vi "Acq Configure Transfer.vi"(0 "session in":refnum<class "Digitizer Control.lvclass">, 1 "host DMA buffer size (samples)":u32[](array[numeric]), 2 "host DMA buffer num of blocks":u32[](array[numeric]), 3 "host DMA buffer block size divisor (bytes)":u32[](array[numeric]), 4 "trigger delay tracking enable (F)":bool, 5 "error in (no error)":errorcluster, 7 "disable DRAM FIFO (F)":bool[](array[boolean]), 9 "enable bit packing (F)":bool[](array[boolean])) -> (13 "sample size (bits)":i32[](array[numeric]), 14 "session out":refnum<class "Digitizer Control.lvclass">, 15 "actual host DMA buffer size (samples)":u32[](array[numeric]), 16 "actual host DMA buffer size (elements)":u32[](array[numeric]), 17 "transfer quantum size (samples)":u64[](array[numeric]), 18 "transfer quantum size (elements)":u64[](array[numeric]), 19 "error out":errorcluster)   [LabVIEW 2021, in "Digitizer Control.lvclass"]
doc: "Configures the acquisition waveform transfer parameters. Note that the transfer parameters can be configured only after the channel parameters are configured. Use the <B>Acq Configure Start Trigger.vi</B> to configure the start trigger, and the <B>Acq Configure Channel.vi</B> to configure the channel parameters. Once the acquisition is configured, use the <B>Acq Initiate.vi</B> to initiate an acquisition, then use the <B>Acq Fetch Waveform.vi</B> to fetch the acquired samples. Use the <B>Acq Get Status.vi</B> to check the acquisition status and the <B>Acq Stop.vi</B> to stop an acquisition.\n\nInputs:\n\n<B>session in</B>: The device session.\n\n<B>host DMA buffer size (samples)</B>: The desired host DMA buffer size given in number of samples. This input is an array, the n-th element corresponds to the n-th channel.\n\n<B>host DMA buffer num of blocks</B>, <B>host DMA buffer block size divisor (bytes)</B>: Use these inputs to apply size constraints on the host DMA buffer size. The size of the allocated host DMA buffer will be a multiple of <B>host DMA buffer num of blocks</B>, and dividing the size of the allocated host DMA buffer by <B>host DMA buffer num of blocks</B> results in a size which is an integer multiple of the sample size, and in bytes is an integer multiple of the <B>host DMA buffer block size divisor (bytes)</B>. These inputs are arrays, the n-th element of an array corresponds to the n-th channel.\n\n<B>trigger delay tracking enable</B>: A true on this input enables the recording of the delay between the device receiving a trigger and starting the acquisition. TClk synchronized acquisitions have an inherent trigger response latency that is between 1-2 TClk periods. The latency can be compensated by acquiring additional pre-trigger samples and keeping only latency worth of the additional pre-trigger samples. When using TClk synchronization, use the <B>Acq Configure Pretrigger Period.vi</B> on all devices to enable the acquisition of the additional pre-trigger samples, and enable this option on the master device to record the trigger response latency. When fetching a record, use the <B>Acq Fetch Trigger Delay.vi</B> on the master device to fetch the recorded delay value and the number of samples to remove from the beginning of the record to align the record with the trigger.\n\n<B>disable DRAM FIFO</B>: Array of booleans, a true in the n-th element of this array disables the use of the DRAM memory available on the device for buffering the samples acquired on the n-th channel.\n\n<B>enable bit packing</B>: Array of booleans, a true in the n-th element of this array enables bit packing for the n-th channel. The device always transfers 16-bit data elements to the host. If bit packing is disabled then the device transfers 16-bit samples to the host, one sample in each data element. If bit packing is enabled then the device transfers 12-bit samples packed into 16-bit data elements to the host (4 samples per 3 data elements).\n\nOutputs:\n\n<B>session out</B>: The device session passed on the <B>session in</B> input.\n\n<B>actual host DMA buffer size (samples)</B>: The actual host DMA buffer size given in number of samples. This output is an array, the n-th element corresponds to the n-th channel.\n\n<B>actual host DMA buffer size (elements)</B>: The actual host DMA buffer size given in number of elements. This output is an array, the n-th element corresponds to the n-th channel.\n\n<B>transfer quantum size (samples)</B>: The smallest number of samples whose size is an integer multiple of the sample transfer interface width. Transferring quantum size multiple samples allows the device to transfer integer number of samples without waiting for further samples to complete the transfer. This output is an array, the n-th element corresponds to the n-th channel.\n\n<B>transfer quantum size (elements)</B>: The number of elements required to transfer <B>transfer quantum size (samples)</B> number of samples. This output is an array, the n-th element corresponds to the n-th channel.\n\n<B>sample size (bits)</B>: The size of a sample, given in bits, the FPGA Target is using when transferring the samples. This output is an array, the n-th element corresponds to the n-th channel."
uses:
  Digitizer Control.lvclass
  Digitizer Control.lvclass/Digitizer Control.ctl
  <vilib>/Utility/error.llb/Error Cluster From Error Code.vi
  <vilib>/rvi/errors/niLvFpgaAdjustHostInterfaceError.vi
  <vilib>/rvi/interface/common/niFpgaWaitOnOcc.vi
  <vilib>/ErrorRing/Error Ring.xnode
  <vilib>/rvi/interface/nirviReadWriteControl/nirviReadWriteControl.xnode
  <vilib>/rvi/interface/nirviMethod/nirviMethod.xnode
  <instrlib>/_niInstr/Streaming/v1/Host/niInstr Streaming v1 Host.lvlib
  <vilib>/rvi/errors/niLvFpgaMergeErrorWithErrorCode.vi
  <vilib>/FPGAPlugInAG/Dynamic/niLvFpga_StartFifo_Dynamic.vi
  <vilib>/FPGAPlugInAG/Dynamic/niLvFpga_ConfigureFifo_Dynamic.vi
  <vilib>/gmath/NI_Gmath.lvlib
  NiFpgaLv.dll
  <vilib>/rvi/interface/Simulation/niFpgaSimulationCallBeginRW.vi
  <vilib>/FPGAPlugInAG/Dynamic/niLvFpga_StopFifo_Dynamic.vi
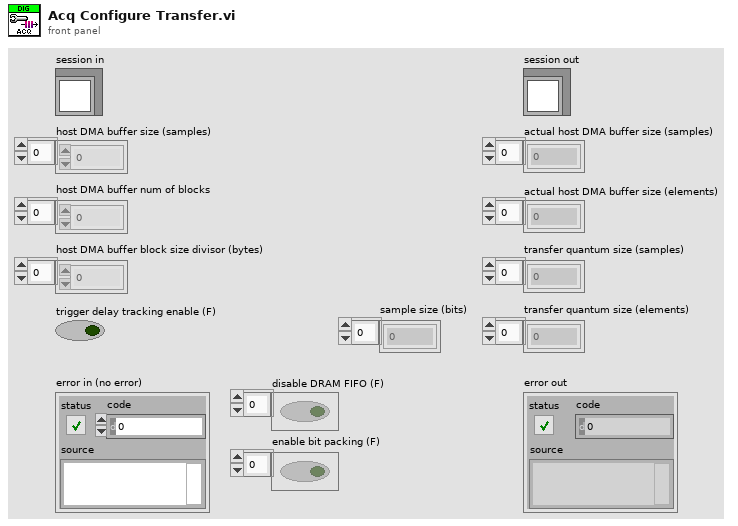
[diagram p1: front panel]
types:
  T1 = typedef "Digitizer Control.lvclass/Acq Session Data.ctl" = cluster{"ADC sampling rate":dbl, "SCTL rate":dbl, "DMA element size (bits)":i32, "sample size (bits)":i32[], "DMA/memory interface width (DMA elements)":i32, "transfer size (bits)":i32[], "stream instance":i32[], "trigger instance":u32, "group delay (s)":dbl, "data delay (s)":dbl, "target delay (s)":dbl, "trigger tracking enabled":bool, "channel configured":bool, "enabled channels":bool[], "transfer configured":bool, "dsp bypass":bool, "fractional decimator input rate":dbl, "fractional decimator output rate":dbl, "sample scale factor":dbl[], "memory size":u64[], "FIFO size":u64}
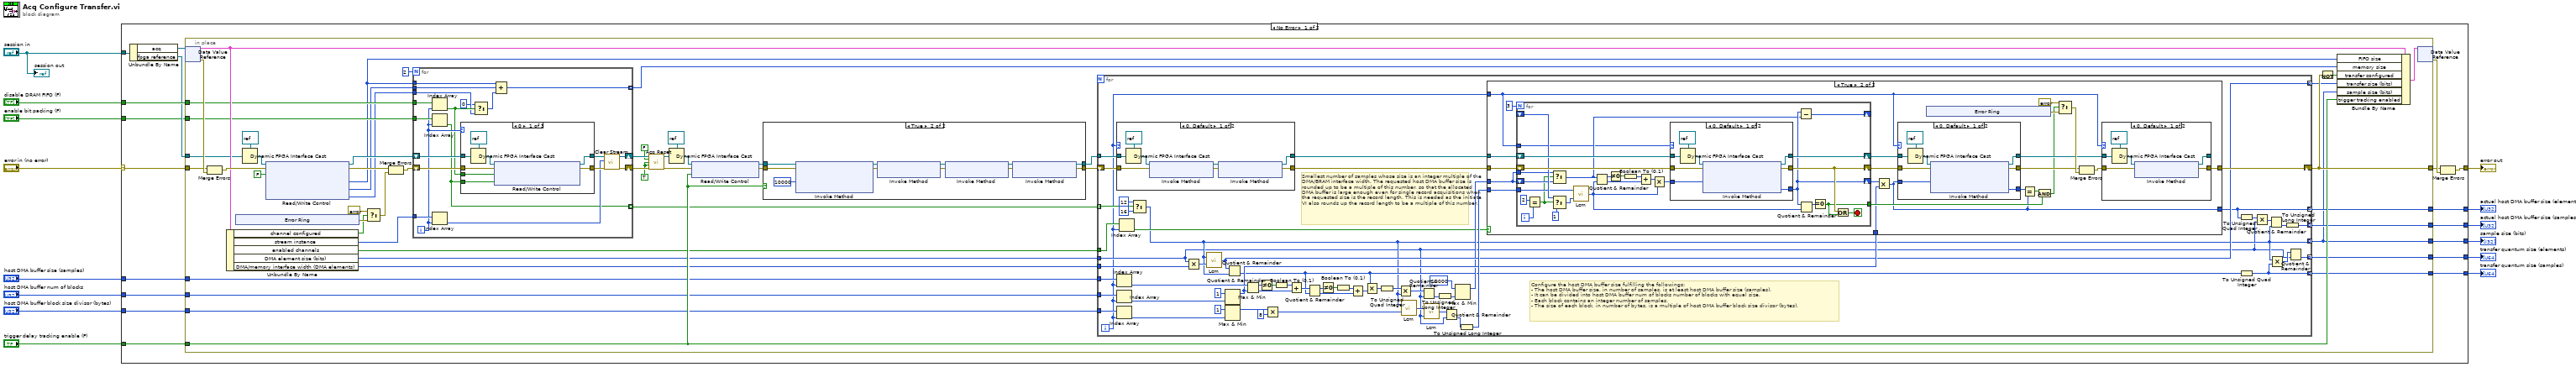
[diagram p0: block diagram]
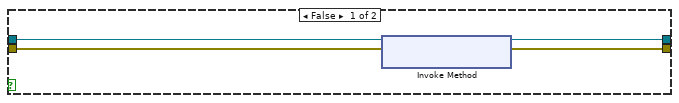
[diagram p2: hidden frame]
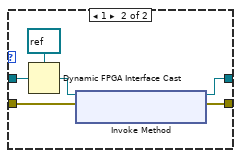
[diagram p4: hidden frame]
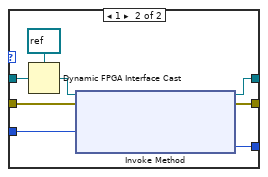
[diagram p5: hidden frame]
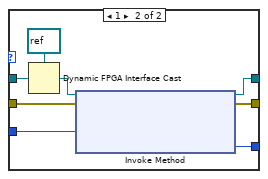
[diagram p6: hidden frame]
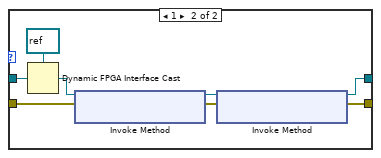
[diagram p7: hidden frame]
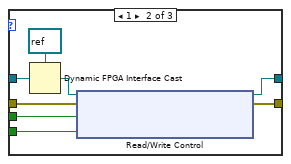
[diagram p8: hidden frame]
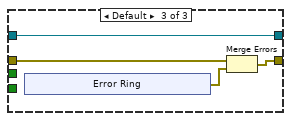
[diagram p9: hidden frame]
diagram:
  n1 = case shown="No Error" "error in (no error)" {
    selector: "error in (no error)" -> [w31 w322]
    tunnel: "session in" -> [w24 _]
    tunnel: [w26 w322] -> w13
    tunnel: "host DMA buffer size (samples)" -> [w30 _]
    tunnel: "disable DRAM FIFO (F)" -> [w29 _]
    tunnel: [w28 _] -> w10
    tunnel: [w25 _] -> w9
    tunnel: "enable bit packing (F)" -> [w21 _]
    tunnel: "trigger delay tracking enable (F)" -> [w20 _]
    tunnel: "host DMA buffer num of blocks" -> [w19 _]
    tunnel: "host DMA buffer block size divisor (bytes)" -> [w18 _]
    tunnel: [w17 _] -> w3
    tunnel: [w16 _] -> w2
    tunnel: [w15 _] -> w1
    frame No Error {
      n2 = Unbundle By Name(w24) -> ("acq"=w23:refnum<data-value>, "fpga reference"=w22:refnum<k20>)
      n3 = in-place {
        in-place-border: [w84] -> w27
        in-place-border: w31 -> [w70]
        in-place-border: w30 -> [w65]
        in-place-border: w29 -> [w42]
        in-place-border: [w66] -> w28
        in-place-border: [w67] -> w25
        in-place-border: w22 -> [w62]
        in-place-border: w21 -> [w59]
        in-place-border: w20 -> [w83]
        in-place-border: w19 -> [w44]
        in-place-border: w18 -> [w43]
        in-place-border: [w36] -> w17
        in-place-border: [w34] -> w16
        in-place-border: [w33] -> w15
        w53 = TRUE
        n4 = in-place-dvr #1(w23) -> (w74:T1, w73:errorcluster)
        n5 = Merge Errors(w70, w73) -> (w79:errorcluster)
        n6 = Unbundle By Name(w74) -> ("channel configured"=w61:bool, "stream instance"=w58:i32[], "enabled channels"=w55:bool[], "DMA element size (bits)"=w63:i32, "DMA/memory interface width (DMA elements)"=w64:i32)
        n7 = xnode "Error Ring"() -> ("error out"=w77:errorcluster)
        n8 = Dynamic FPGA Interface Cast(Session In=refnum<k20> refnum ("FPGA Interface"), Type=w62) -> (Session Out=w71:refnum<k20>)
        n9 = xnode "Read/Write Control"("FPGA VI Reference In"=w71, "error in"=w79, "acq.stream.start enable"=FALSE) -> ("FPGA VI Reference Out"=w60:refnum<k20>, "error out"=w78:errorcluster, "acq.wfm.FIFO size"=w38:u64, "acq.wfm.memory FIFO size"=w40:u64, "acq.wfm.memory DRAM size"=w39:u64)
        n10 = Select(t=errorcluster {"status"=FALSE, "code"=0, "source"=""}, s=w61, f=w77) -> (s? t:f=w75:errorcluster)
        n11 = Merge Errors(w78, w75) -> (w80:errorcluster)
        n12 = for {
          N: 2 -> [_]
          tunnel: w59 -> [w287]
          tunnel: w42 -> [w286]
          tunnel: w58 -> [w285]
          shift-right: [w291] -> w81
          shift-left: w80 -> [w289]
          tunnel: [w280] -> w56 mode=indexing
          shift-right: [w284] -> w82
          shift-left: w60 -> [w288]
          tunnel: w40 -> [w275]
          tunnel: w39 -> [w278]
          tunnel: w38 -> [w276]
          tunnel: [w273] -> w37 mode=indexing
          i -> [w281]
          n13 = Index Array(array=w286, index=w281) -> (element=w279:bool)
          n14 = Index Array(array=w287, index=w281) -> (element=w280:bool)
          n15 = Index Array(array=w285, index=w281) -> (element=w282:i32)
          n16 = case shown="0" w281 {
            tunnel: w288 -> [w297 w307 w311]
            tunnel: w289 -> [w299 w306 w310]
            tunnel: w279 -> [w296 w305 _]
            tunnel: w280 -> [w295 w304 _]
            tunnel: [w298 w301 w309] -> w290
            tunnel: [w292 w300 w311] -> w283
            frame 0 {
              n17 = Dynamic FPGA Interface Cast(Session In=refnum<k20> refnum ("FPGA Interface"), Type=w297) -> (Session Out=w293:refnum<k20>)
              n18 = xnode "Read/Write Control"("FPGA VI Reference In"=w293, "error in"=w299, "acq.wfm.bypass DRAM FIFO 0"=w296, "acq.wfm.enable bit packing 0"=w295) -> ("FPGA VI Reference Out"=w292:refnum<k20>, "error out"=w298:errorcluster)
            }
            frame 1 {
              n19 = Dynamic FPGA Interface Cast(Session In=refnum<k20> refnum ("FPGA Interface"), Type=w307) -> (Session Out=w302:refnum<k20>)
              n20 = xnode "Read/Write Control"("FPGA VI Reference In"=w302, "error in"=w306, "acq.wfm.bypass DRAM FIFO 1"=w305, "acq.wfm.enable bit packing 1"=w304) -> ("FPGA VI Reference Out"=w300:refnum<k20>, "error out"=w301:errorcluster)
            }
            frame Default {
              n21 = xnode "Error Ring"() -> ("error out"=w308:errorcluster)
              n22 = Merge Errors(w310, w308) -> (w309:errorcluster)
            }
          }
          n23 = Select(t=u64 0, s=w279, f=w278) -> (s? t:f=w274:u64)
          n24 = Compound Arithmetic op=ADD(w276, w275, w274) -> (w273:u64)
          n25 = call <instrlib>:"Clear Stream.vi"("error in (no error)"=w290, "stream index"=w282, "refnum in"=w283) -> ("error out"=w291:errorcluster, "refnum out"=w284:refnum<k20>)  [unwired: 7 in]
        }
        n26 = call "Acq Reset.vi"("fpga reference in"=w82, "reset dsp"=FALSE, "reset stream control"=w53, "reset waveform streaming"=w53, "error in (no error)"=w81) -> ("fpga reference out"=w49:refnum<k20>, "error out"=w48:errorcluster)  [unwired: 9 in]
        n27 = Dynamic FPGA Interface Cast(Session In=refnum<k20> refnum ("FPGA Interface"), Type=w49) -> (Session Out=w47:refnum<k20>)
        n28 = xnode "Read/Write Control"("FPGA VI Reference In"=w47, "error in"=w48, "trigger.monitor enable"=w83) -> ("FPGA VI Reference Out"=w45:refnum<k20>, "error out"=w46:errorcluster)
        n29 = case shown="True" w83 {
          tunnel: w46 -> [w88 w99]
          tunnel: [w85 w90] -> w52
          tunnel: w45 -> [w87 w97]
          tunnel: [w86 w89] -> w51
          frame False {
            n30 = xnode "Invoke Method"("FPGA VI Reference In"=w87, "error in"=w88) -> ("FPGA VI Reference Out"=w86:refnum<k20>, "error out"=w85:errorcluster)
          }
          frame True {
            n31 = xnode "Invoke Method"("FPGA VI Reference In"=w97, "error in"=w99, "Requested Depth"=u32 10000) -> ("FPGA VI Reference Out"=w95:refnum<k20>, "error out"=w96:errorcluster)  [unwired: 1 out]
            n32 = xnode "Invoke Method"("FPGA VI Reference In"=w95, "error in"=w96) -> ("FPGA VI Reference Out"=w93:refnum<k20>, "error out"=w94:errorcluster)
            n33 = xnode "Invoke Method"("FPGA VI Reference In"=w93, "error in"=w94) -> ("FPGA VI Reference Out"=w91:refnum<k20>, "error out"=w92:errorcluster)
            n34 = xnode "Invoke Method"("FPGA VI Reference In"=w91, "error in"=w92) -> ("FPGA VI Reference Out"=w89:refnum<k20>, "error out"=w90:errorcluster)
          }
        }
        n35 = for {
          tunnel: [w154] -> w67 mode=indexing
          tunnel: [w112] -> w66 mode=indexing
          tunnel: w65 -> [w153]
          tunnel: w64 -> [w152]
          tunnel: w63 -> [w102]
          tunnel: [w114] -> w35 mode=indexing
          tunnel: w56 -> [w121] mode=indexing
          tunnel: [w104] -> w34 mode=indexing
          tunnel: w55 -> [w119]
          shift-right: [w157] -> w84
          shift-left: w52 -> [w155]
          tunnel: w51 -> [w156]
          tunnel: w44 -> [w110]
          tunnel: w43 -> [w108]
          tunnel: [w105] -> w36 mode=indexing
          tunnel: [w101] -> w33 mode=indexing
          i -> [w100]
          # "Smallest number of samples whose size is an integer multiple of the DMA/BRAM interface width. The requested host DMA buffer size is rounded up to be a multiple of this number, so that the allocated DMA buffer is large enough even for single record acquisitions when the requested size is the record length. This is needed as the initiate VI also rounds up the record length to be a multiple of this number."
          # "Configure the host DMA buffer size fulfilling the followings:\n- The host DMA buffer size, in number of samples, is at least host DMA buffer size (samples).\n- It can be divided into host DMA buffer num of blocks number of blocks with equal size.\n- Each block contains an integer number of samples.\n- The size of each block, in number of bytes, is a multiple of host DMA buffer block size divisor (bytes)."
          n36 = case shown="0, Default" w100 {
            tunnel: [w262 w270] -> w125
            tunnel: [w261 w269] -> w124
            tunnel: w156 -> [w258 w266]
            tunnel: w155 -> [w260 w268]
            frame 0, Default {
              n37 = Dynamic FPGA Interface Cast(Session In=refnum<k20> refnum ("FPGA Interface"), Type=w258) -> (Session Out=w257:refnum<k20>)
              n38 = xnode "Invoke Method"("FPGA VI Reference In"=w257, "error in"=w260) -> ("FPGA VI Reference Out"=w263:refnum<k20>, "error out"=w264:errorcluster)
              n39 = xnode "Invoke Method"("FPGA VI Reference In"=w263, "error in"=w264) -> ("FPGA VI Reference Out"=w261:refnum<k20>, "error out"=w262:errorcluster)
            }
            frame 1 {
              n40 = Dynamic FPGA Interface Cast(Session In=refnum<k20> refnum ("FPGA Interface"), Type=w266) -> (Session Out=w265:refnum<k20>)
              n41 = xnode "Invoke Method"("FPGA VI Reference In"=w265, "error in"=w268) -> ("FPGA VI Reference Out"=w271:refnum<k20>, "error out"=w272:errorcluster)
              n42 = xnode "Invoke Method"("FPGA VI Reference In"=w271, "error in"=w272) -> ("FPGA VI Reference Out"=w269:refnum<k20>, "error out"=w270:errorcluster)
            }
          }
          n43 = Index Array(array=w153, index=w100) -> (element=w123:u32)
          n44 = Index Array(array=w110, index=w100) -> (element=w109:u32)
          n45 = Index Array(array=w108, index=w100) -> (element=w107:u32)
          n46 = Index Array(array=w119, index=w100) -> (element=w111:bool)
          n47 = Select(t=12, s=w121, f=16) -> (s? t:f=w104:i32)
          n48 = Multiply(x=w102, y=w152) -> (x*y=w136:i32)
          n49 = call <vilib>:"Lcm.vi"("y"=w136, "x"=w104) -> ("lcm(x,y)"=w114:i64)
          n50 = Max & Min(x=u32 1, y=w109) -> (max(x,y)=w118:u32)  [unwired: 1 out]
          n51 = Max & Min(x=u32 1 ("y"), y=w107) -> (max(x,y)=w117:u32)  [unwired: 1 out]
          n52 = Quotient & Remainder(x=w114, y=w104) -> (floor(x/y)=w106:i64)  [unwired: 1 out]
          n53 = Quotient & Remainder(x=w123, y=w118) -> (x-y*floor(x/y)=w140:u32, floor(x/y)=w137:u32)
          n54 = Not Equal To 0?(x=w140) -> (x != 0?=w139:bool)
          n55 = Multiply(x=w117, y=u32 8) -> (x*y=w149:u32)
          n56 = Boolean To (0,1)(Boolean=w139) -> (0, 1=w138:i16)
          n57 = Add(x=w138, y=w137) -> (x+y=w130:u32)
          n58 = Quotient & Remainder(x=w130, y=w106) -> (x-y*floor(x/y)=w131:i64, floor(x/y)=w134:i64)
          n59 = Not Equal To 0?(x=w131) -> (x != 0?=w132:bool)
          n60 = Boolean To (0,1)(Boolean=w132) -> (0, 1=w133:i16)
          n61 = Add(x=w133, y=w134) -> (x+y=w135:i64)
          n62 = Multiply(x=w106, y=w135) -> (x*y=w129:i64)
          n63 = To Unsigned Quad Integer(1:w129) -> (0:w128:u64)
          n64 = Multiply(x=w128, y=w104) -> (x*y=w146:u64)
          n65 = call <vilib>:"Lcm.vi"("y"=w149, "x"=w104) -> ("lcm(x,y)"=w148:i64)
          n66 = Quotient & Remainder(x=w146, y=w102) -> (floor(x/y)=w127:u64)  [unwired: 1 out]
          n67 = call <vilib>:"Lcm.vi"("y"=w102, "x"=w148) -> ("lcm(x,y)"=w147:i64)
          n68 = To Unsigned Long Integer(number=w127) -> (unsigned 32bit integer=w126:u32)
          n69 = Quotient & Remainder(x=w147, y=w102) -> (floor(x/y)=w141:i64)  [unwired: 1 out]
          n70 = Max & Min(x=u32 10000, y=w126) -> (max(x,y)=w113:u32)  [unwired: 1 out]
          n71 = To Unsigned Long Integer(number=w141) -> (unsigned 32bit integer=w145:u32)
          n72 = case shown="True" w111 {
            tunnel: w145 -> [_ w174]
            tunnel: w125 -> [w158 w170]
            tunnel: w124 -> [_ w169]
            tunnel: w118 -> [_ w168]
            tunnel: w113 -> [_ w167]
            tunnel: [_ w162] -> w112
            tunnel: [w158 w161] -> w157
            tunnel: w100 -> [_ w159]
            frame False {
            }
            frame True {
              n73 = for {
                N: 3 -> [_]
                shift-right: [w239] -> w164
                shift-left: w169 -> [w237]
                shift-right: [w240] -> w165
                shift-left: w170 -> [w238]
                tunnel: w174 -> [w223]
                tunnel: [w236] -> w171
                shift-right: [w229] -> w173
                shift-left: w167 -> [w219]
                shift-right: [w228] -> _
                shift-left: _ -> [w226]
                tunnel: w167 -> [w216]
                tunnel: w159 -> [w215]
                i -> [w221]
                stop <- w214 stop-if-true
                n74 = Equal?(x=2, y=w221) -> (x = y?=w218:bool)
                n75 = Select(t=w216, s=w218, f=w219) -> (s? t:f=w217:u32)
                n76 = Select(t=w226, s=w218, f=u32 1) -> (s? t:f=w224:u32)
                n77 = call <vilib>:"Lcm.vi"("y"=w224, "x"=w223) -> ("lcm(x,y)"=w222:i64)
                n78 = Quotient & Remainder(x=w217, y=w222) -> (x-y*floor(x/y)=w235:i64, floor(x/y)=w232:i64)
                n79 = Not Equal To 0?(x=w235) -> (x != 0?=w234:bool)
                n80 = Boolean To (0,1)(Boolean=w234) -> (0, 1=w233:i16)
                n81 = Add(x=w233, y=w232) -> (x+y=w231:i64)
                n82 = Multiply(x=w231, y=w222) -> (x*y=w230:i64)
                n83 = case shown="0, Default" w215 {
                  tunnel: w238 -> [w248 w256]
                  tunnel: [w247 w255] -> w240
                  tunnel: [w246 w254] -> w239
                  tunnel: w237 -> [w242 w250]
                  tunnel: w230 -> [w245 w253]
                  tunnel: [w244 w252] -> w229
                  frame 0, Default {
                    n84 = Dynamic FPGA Interface Cast(Session In=refnum<k20> refnum ("FPGA Interface"), Type=w242) -> (Session Out=w241:refnum<k20>)
                    n85 = xnode "Invoke Method"("FPGA VI Reference In"=w241, "error in"=w248, "Requested Depth"=w245) -> ("FPGA VI Reference Out"=w246:refnum<k20>, "error out"=w247:errorcluster, "Actual Depth"=w244:u32)
                  }
                  frame 1 {
                    n86 = Dynamic FPGA Interface Cast(Session In=refnum<k20> refnum ("FPGA Interface"), Type=w250) -> (Session Out=w249:refnum<k20>)
                    n87 = xnode "Invoke Method"("FPGA VI Reference In"=w249, "error in"=w256, "Requested Depth"=w253) -> ("FPGA VI Reference Out"=w254:refnum<k20>, "error out"=w255:errorcluster, "Actual Depth"=w252:u32)
                  }
                }
                n88 = Subtract(x=w229, y=w217) -> (x-y=w228:u32)
                n89 = Quotient & Remainder(x=w229, y=w222) -> (x-y*floor(x/y)=w220:i64)  [unwired: 1 out]
                n90 = Equal To 0?(x=w220) -> (x = 0?=w236:bool)
                n91 = Or(x=w240, y=w236) -> (x .or. y?=w214:bool)
              }
              n92 = Multiply(x=w173, y=w168) -> (x*y=w162:u32)
              n93 = case shown="0, Default" w159 {
                tunnel: w165 -> [w200 w208]
                tunnel: [w199 w207] -> w177
                tunnel: [w198 w206] -> w176
                tunnel: w164 -> [w195 w202]
                tunnel: w162 -> [w193 w205]
                tunnel: [w197 w204] -> w163
                frame 0, Default {
                  n94 = Dynamic FPGA Interface Cast(Session In=refnum<k20> refnum ("FPGA Interface"), Type=w195) -> (Session Out=w194:refnum<k20>)
                  n95 = xnode "Invoke Method"("FPGA VI Reference In"=w194, "error in"=w200, "Requested Depth"=w193) -> ("FPGA VI Reference Out"=w198:refnum<k20>, "error out"=w199:errorcluster, "Actual Depth"=w197:u32)
                }
                frame 1 {
                  n96 = Dynamic FPGA Interface Cast(Session In=refnum<k20> refnum ("FPGA Interface"), Type=w202) -> (Session Out=w201:refnum<k20>)
                  n97 = xnode "Invoke Method"("FPGA VI Reference In"=w201, "error in"=w208, "Requested Depth"=w205) -> ("FPGA VI Reference Out"=w206:refnum<k20>, "error out"=w207:errorcluster, "Actual Depth"=w204:u32)
                }
              }
              n98 = xnode "Error Ring"() -> ("error out"=w180:errorcluster)
              n99 = Equal?(x=w163, y=w162) -> (x = y?=w172:bool)
              n100 = And(x=w172, y=w171) -> (x .and. y?=w166:bool)
              n101 = Select(t=errorcluster {"status"=FALSE, "code"=0, "source"=""}, s=w166, f=w180) -> (s? t:f=w178:errorcluster)
              n102 = Merge Errors(w177, w178) -> (w160:errorcluster)
              n103 = case shown="0, Default" w159 {
                tunnel: w160 -> [w186 w192]
                tunnel: [w185 w191] -> w161
                tunnel: [w184 w190] -> _
                tunnel: w176 -> [w182 w188]
                frame 0, Default {
                  n104 = Dynamic FPGA Interface Cast(Session In=refnum<k20> refnum ("FPGA Interface"), Type=w182) -> (Session Out=w181:refnum<k20>)
                  n105 = xnode "Invoke Method"("FPGA VI Reference In"=w181, "error in"=w186) -> ("FPGA VI Reference Out"=w184:refnum<k20>, "error out"=w185:errorcluster)
                }
                frame 1 {
                  n106 = Dynamic FPGA Interface Cast(Session In=refnum<k20> refnum ("FPGA Interface"), Type=w188) -> (Session Out=w187:refnum<k20>)
                  n107 = xnode "Invoke Method"("FPGA VI Reference In"=w187, "error in"=w192) -> ("FPGA VI Reference Out"=w190:refnum<k20>, "error out"=w191:errorcluster)
                }
              }
            }
          }
          n108 = To Unsigned Quad Integer(1:w112) -> (0:w144:u64)
          n109 = To Unsigned Quad Integer(1:w106) -> (0:w105:u64)
          n110 = Multiply(x=w144, y=w102) -> (x*y=w143:u64)
          n111 = Quotient & Remainder(x=w143, y=w104) -> (floor(x/y)=w142:u64)  [unwired: 1 out]
          n112 = Multiply(x=w104, y=w105) -> (x*y=w103:u64)
          n113 = To Unsigned Long Integer(number=w142) -> (unsigned 32bit integer=w154:u32)
          n114 = Quotient & Remainder(x=w103, y=w102) -> (floor(x/y)=w101:u64)  [unwired: 1 out]
        }
        n115 = Not(x=w84) -> (.not. x?=w41:bool)
        n116 = Bundle By Name(cluster=w74, "FIFO size"=w38, "memory size"=w37, "transfer configured"=w41, "transfer size (bits)"=w35, "sample size (bits)"=w34, "trigger tracking enabled"=w83) -> (w69:T1)
        n117 = in-place-dvr #1(w69) -> (w32:errorcluster)  [unwired: 1 out]
      }
      n118 = Merge Errors(w27, w32) -> (w26:errorcluster)
    }
    frame Error {
    }
  }
  "error out" <- w13
  "actual host DMA buffer size (elements)" <- w10
  "actual host DMA buffer size (samples)" <- w9
  "transfer quantum size (samples)" <- w3
  "sample size (bits)" <- w2
  "transfer quantum size (elements)" <- w1
  "session out" <- "session in"
